vi "SrsQcm200GetResistance.vi"(0 "VISA in":refnum<visa-resource-name>, 5 "error in (no error)":errorcluster) -> (14 "VISA out":refnum<visa-resource-name>, 17 "Resistance out":dbl format="%.6e", 19 "error out":errorcluster)   [LabVIEW 2013]
doc: "This VI queries the loss of the circuit driving the QCM200 oscillation. The value is returned in ohms.\n\nCopyright 2003 Stanford Research Systems. All rights reserved."
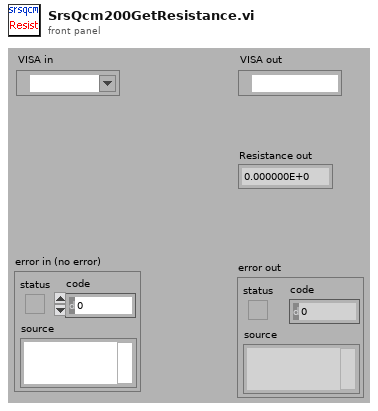
[diagram p1: front panel]
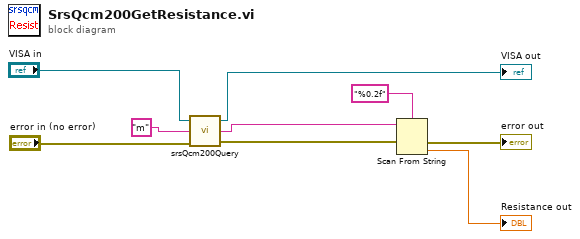
[diagram p0: block diagram]
diagram:
  n1 = call <instrlib>:"srsQcm200Query.vi"("error in"="error in (no error)", "Command"="m" ("write buffer (\"\")"), "VISA in"="VISA in") -> ("error out"=w2:errorcluster, "Output"=w1:string, "VISA out"=→"VISA out":refnum<visa-resource-name>)
  n2 = Scan From String(format string="%0.2f", input string=w1, error in=w2) -> (error out=→"error out":errorcluster, output 1=→"Resistance out":dbl)  [unwired: 2 in, 2 out]
